vi "BinMLE.vi"(0 "channel width (ns)":dbl format="%.2f", 1 "channel count":i32, 3 "rebinning":i32, 4 "binning":dbl format="%.2f", 5 "input range":cluster{"x0":dbl, "x1":dbl} {"x1" format="%.2f"; "x0" format="%.2f"}, 6 "rawdata":T1) -> (2 "MLE trace":dbl[](array[numeric]) format="%.2f")   [LabVIEW 2009]
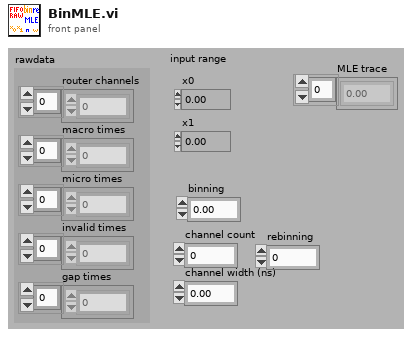
[diagram p1: front panel]
types:
  T1 = cluster{"router channels":u8[], "macro times":u32[], "micro times":u16[], "invalid times":u32[], "gap times":u32[]}
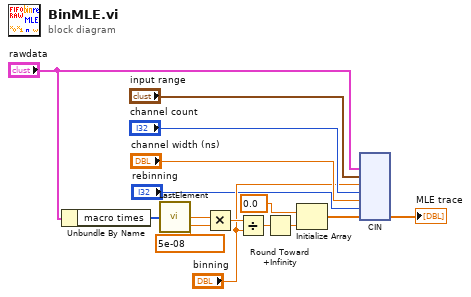
[diagram p0: block diagram]
diagram:
  n1 = Unbundle By Name("rawdata") -> ("macro times"=w5:u32[])
  n2 = call "LastElement.vi"("array"=w5) -> ("Numeric"=w9:dbl)
  n3 = Multiply(x=w9, y=5e-08) -> (x*y=w12:dbl)
  n4 = Divide(x=w12, y="binning") -> (x/y=w13:dbl)
  n5 = Round Toward +Infinity(x=w13) -> (ceil(x): smallest int >= x=w1:dbl)
  n6 = Initialize Array(0.0 ("element"), w1) -> (w14:dbl[])
  n7 = cin("rawdata", "input range", "binning", "channel count", "channel width (ns)", "rebinning", w14) -> (→"MLE trace":dbl[])  [unwired: 6 in]
